vi "set_flexray_ub_bit_auto_handle.vi"(8 "error in (no error)":errorcluster caption="错误输入（无错误）", 10 "AIsAutoHandle":bool, 11 "path in":path) -> (0 "error out":errorcluster caption="错误输出", 2 "function return":i32, 3 "path out":path)   [LabVIEW 2014]
doc: "TSAPI(s32)set_flexray_ub_bit_auto_handle(const bool AIsAutoHandle);"
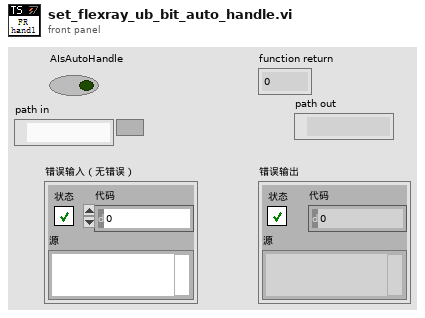
[diagram p1: front panel]
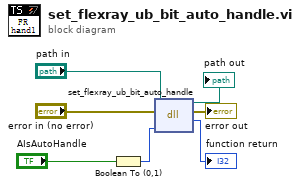
[diagram p0: block diagram]
diagram:
  n1 = Boolean To (0,1)(Boolean="AIsAutoHandle") -> (0, 1=w5:i16)
  n2 = dll-call lib="D:/Work/LabVIEW Code/TSMaster Labview SDK/LabVIEW/LabVIEW-TSMasterAPI_CLN/TSMasterAPI_LabVIEW-2024-10-08 14-20-13/Not_organized_vi/TSMaster.*" fn="set_flexray_ub_bit_auto_handle"(path in="path in", error in="error in (no error)", "AIsAutoHandle"=w5) -> (path out=→"path out":path, error out=→"error out":errorcluster, "返回类型"=→"function return":i32)  [unwired: 2 in]
